vi "Write.vi"(8 "error in (no error)":errorcluster, 9 "Connection Name":string, 11 "Command":string) -> (0 "error out":errorcluster, 3 "Return String":string)   [LabVIEW 2015, in "LabSSH.lvlib"]
doc: "<License>This software is distributed under the BSD 3-Clause License. For the full license please see license.txt or visit www.labvolution.com/license</License>"
uses:
  LabSSH.lvlib
  FGV State..enum.ctl
  C:/Working Folder/ssh.git/LabSSH Library/References/LabSSH.dll
  References/LabSSH.dll
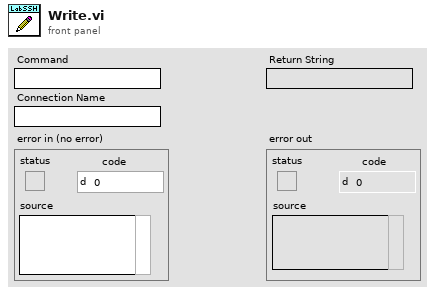
[diagram p1: front panel]
types:
  T1 = typedef "LabSSH.lvlib/FGV State..enum.ctl" = enum16{"GET", "SET"}
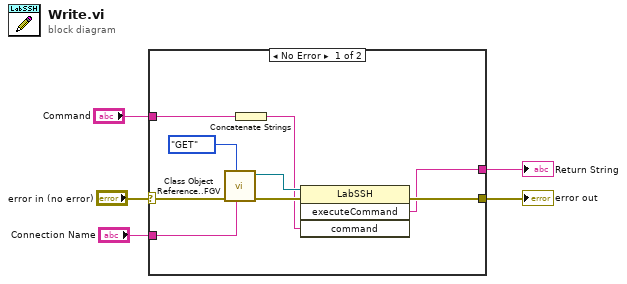
[diagram p0: block diagram]
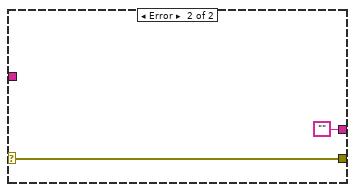
[diagram p2: hidden frame]
diagram:
  n1 = case shown="No Error" "error in (no error)" {
    selector: "error in (no error)" -> [w14 w16]
    tunnel: [w10 w16] -> w4
    tunnel: [w9 ""] -> w3
    tunnel: "Command" -> [w8 _]
    tunnel: "Connection Name" -> [w6 _]
    frame No Error {
      n2 = call "Class Object Reference..FGV.vi"("Connection Name"=w6, "FGV State (GET)"=FGV_State..enum."GET" ("FGV State"), "error in (no error)"=w14) -> ("error out"=w11:errorcluster, "LabSSH ref out"=w12:refnum<k24>)  [unwired: 7 in]
      n3 = Concatenate Strings(w8) -> (w7:string)
      n4 = invoke class="LabSSH" method="executeCommand"(reference=w12, error in=w11, "command"=w7) -> (error out=w10:errorcluster, "executeCommand"=w9:string)  [unwired: 1 in, 2 out]
    }
    frame Error {
    }
  }
  "error out" <- w4
  "Return String" <- w3
